vi "Configure PID.vi"(0 "VISA resource name":refnum<visa-resource-name>, 5 "Output's Control Loop (1:1)":u16(ring)=1 items=["1"=1, "2"=2], 7 "Gain (P) (50.0)":dbl=50.0 format="%.1f", 9 "Reset (I) (20.0)":dbl=20.0 format="%.1f", 11 "error in (no error)":errorcluster, 12 "Rate (D) (0.0 %)":dbl format="%.1f") -> (4 "VISA resource name out":refnum<visa-resource-name>, 15 "error out":errorcluster)   [LabVIEW 2019, in "Lake Shore 335.lvlib"]
doc: "Configures the Proportional (P), Integral (I), and Derivative (D) control parameters. Control settings (P, I, D, and Setpoint) are assigned to heater outputs, which results in the settings being applied to any loop formed by the output and its control input."
uses:
  Lake Shore 335.lvlib
  Instance           1 21Saved   Configure PID .vi
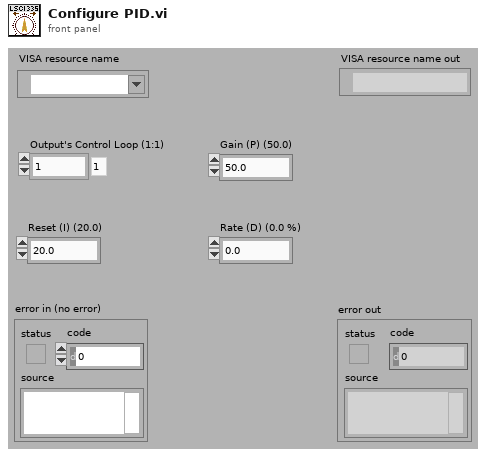
[diagram p1: front panel]
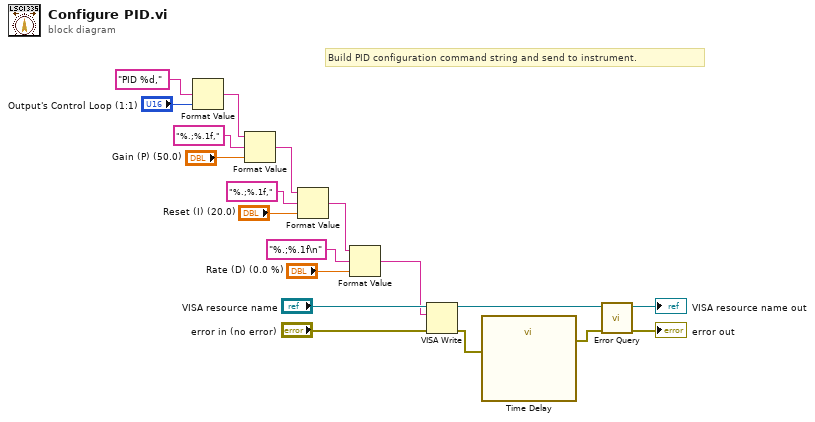
[diagram p0: block diagram]
diagram:
  # "Build PID configuration command string and send to instrument."
  n1 = Format Value(format string="PID %d,", value (0)="Output's Control Loop (1:1)") -> (output string=w1:string)  [unwired: 1 in]
  n2 = Format Value(string ("")=w1, format string="%.;%.1f,", value (0)="Gain (P) (50.0)") -> (output string=w8:string)
  n3 = Format Value(string ("")=w8, format string="%.;%.1f,", value (0)="Reset (I) (20.0)") -> (output string=w7:string)
  n4 = Format Value(string ("")=w7, format string="%.;%.1f\n", value (0)="Rate (D) (0.0 %)") -> (output string=w4:string)
  n5 = VISA Write(VISA resource name="VISA resource name", write buffer=w4, error in (no error)="error in (no error)") -> (VISA resource name out=w17:refnum<visa-resource-name>, error out=w14:errorcluster)  [unwired: 1 out]
  n6 = call "Time Delay"("error in (no error)"=w14) -> ("error out"=w13:errorcluster)  [unwired: 10 in]
  n7 = call "Error Query.vi"("error in (no error)"=w13, "VISA resource name"=w17) -> ("error out"=→"error out":errorcluster, "VISA resource name out"=→"VISA resource name out":refnum<visa-resource-name>)  [unwired: 7 in, 1 out]
